vi "Assert Is Class.vi"(5 "Assert Only? (F)":bool, 6 "error code (1)":i32=1, 7 "Label":string="Class is correct", 8 "Error In":errorcluster, 10 "Expected":refnum<class>, 11 "Actual":refnum<class>) -> (0 "Error Out":errorcluster)   [LabVIEW 2017, in "Tests.lvlib"]
uses:
  Tests.lvlib
  <vilib>/addons/_JKI Toolkits/Caraya/classes/Assert/Assert.lvclass
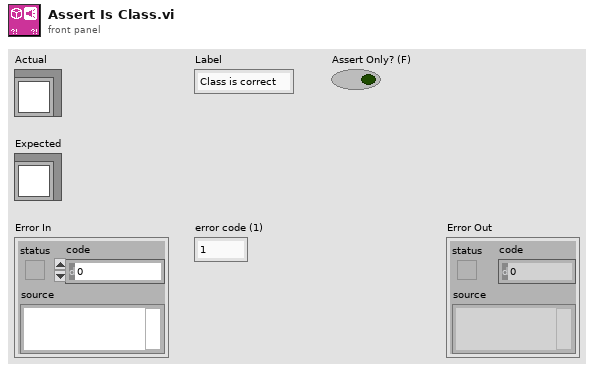
[diagram p1: front panel]
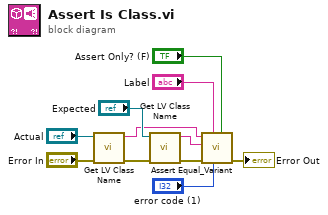
[diagram p0: block diagram]
diagram:
  n1 = call <vilib>:"Get LV Class Name.vi"("error in (no error)"="Error In", "object"="Actual") -> ("error out"=w9:errorcluster, "class name"=w6:string)  [unwired: 8 in]
  n2 = call <vilib>:"Get LV Class Name.vi"("error in (no error)"=w9, "object"="Expected") -> ("error out"=w7:errorcluster, "class name"=w5:string)  [unwired: 8 in]
  n3 = call <vilib>:"Assert Equal_Variant.vi"("Assert Only? (F)"="Assert Only? (F)", "error code (1)"="error code (1)", "Label"="Label", "error in (no error)"=w7, "Y"=w5, "X"=w6) -> ("error out"=→"Error Out":errorcluster)  [unwired: 5 in]
